vi "download.vi"   [LabVIEW 2015, in "lv-dropbox.lvlib" / "v2.lvlib"]
uses:
  v2.lvlib
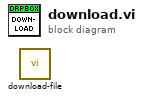
[diagram p0: block diagram]
diagram:
  n1 = call "download-file.vi"() -> ()  [unwired: 11 in, 1 out]
